vi "Dashboard Main.vi"() -> ()   [LabVIEW 2018]
uses:
  <vilib>/Rock Robotics/Network Tables/NT Read Numeric Array.vi
panel:
  out "Camera Perf":string
  in  "Camera Settings":T1={"Frame Rate"=30, "Compression"=30, "Size"=1, "DB Camera Config"=FALSE} {"Frame Rate" scale=1.0..30.0; "Compression" scale=100.0..-1.0; "Size" items=["640x480", "320x240", "160x120"]}
  in  "TCP":refnum<k5>
  out "Robot IP":string
  in  "Dashboard Tab":enum32{"Drive", "Basic", "Custom", "Variables"}(tab)
  in  "Select Auto":string(combo)="Select Autonomous ..."
  out "NT Connection":bool
  out "MotorChart R":cluster{"Numeric":dbl, "Numeric":dbl}(graph)
  out "MotorChart L":cluster{"Numeric":dbl, "Numeric":dbl}(graph)
  out "MotorSliders R":cluster{"MotorSlide1":dbl, "MotorSlide2":dbl} {"MotorSlide2" scale=-1.0..1.0 scale format="%#_2e"; "MotorSlide1" scale=-1.0..1.0 scale format="%#_2e"}
  out "MotorSliders L":cluster{"MotorSlide1":dbl, "MotorSlide2":dbl} {"MotorSlide2" scale=-1.0..1.0 scale format="%#_2e"; "MotorSlide1" scale=-1.0..1.0 scale format="%#_2e"}
  out "JS1 Z":dbl(slide) scale=-1.0..1.0 scale format="%#_2e"
  out "JS1 Graph":cluster{"X":dbl, "Y":dbl}[](graph)
  out "JS1 Buttons":T2
  out "JS2 Z":dbl(slide) scale=-1.0..1.0 scale format="%#_2e"
  out "JS2 Graph":cluster{"X":dbl, "Y":dbl}[](graph)
  out "JS2 Buttons":T2
  out "Mode":T3(ring)=enum."Auto Disabled"
  in  "DB/String 9":string
  in  "DB/String 8":string
  in  "DB/String 7":string
  in  "DB/String 6":string
  in  "DB/String 5":string
  in  "DB/String 4":string
  in  "DB/String 3":string
  in  "DB/String 2":string
  in  "DB/String 1":string
  in  "DB/String 0":string
  in  "DB/Slider 0":dbl(slide) scale=0.0..5.0
  in  "DB/Slider 1":dbl(slide) scale=0.0..5.0
  in  "DB/Slider 2":dbl(slide) scale=0.0..5.0
  in  "DB/Slider 3":dbl(slide) scale=0.0..5.0
  out "DB/LED 3":bool
  out "DB/LED 2":bool
  out "DB/LED 1":bool
  out "DB/LED 0":bool
  in  "DB/Button 3":bool
  in  "DB/Button 2":bool
  in  "DB/Button 1":bool
  in  "DB/Button 0":bool caption="New Name"
  out "Tree":string(tree)
  out "Camera Image":T4(plugin-control)
  out "Background":bool
  in  "Camera Name":string(combo)="No Camera Selection"
  # "HW"
  # "Joysticks"
  # "Drive Motors"
  # "Front"
  # "Right"
  # "Left"
  # "Back"
  # "This tab is a great place for autonomous settings and robot-specific values.\nPlace controls and indicators inside this tab and match name to\nDashboard Variables on robot. You can also delete this comment."
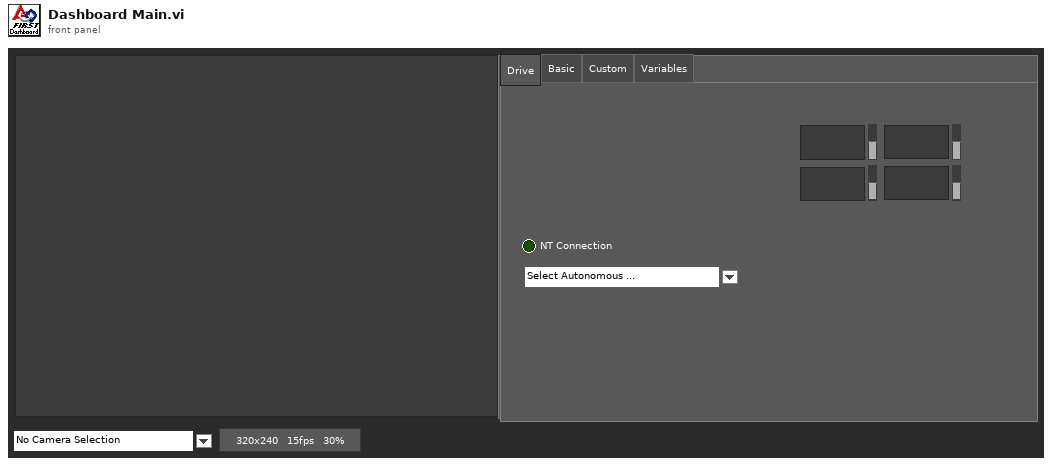
[diagram p1: front panel]
types:
  T1 = cluster{"Frame Rate":i32, "Compression":i32, "Size":u16, "DB Camera Config":bool}
  T2 = cluster{bool, bool, bool, bool, bool, bool, bool, bool, bool, bool, bool, bool}
  T3 = enum8{"Tele-Op Disabled", "Tele-Op Enabled", "Auto Disabled", "Auto Enabled", "Test Disabled", "Test Enabled", "Disconnected", "No Code", "E-Stop"}
  T4 = typedef "IMAQ Image.ctl" = refnum<image>
  T5 = cluster{"Save Path":path, "Interval (s)":dbl, "Keep":i32}
  T6 = typedef "Image Type" = u32
  T7 = cluster{"Camera Image":refnum<vi>, "Dashboard Tab":refnum<vi>, "Background":refnum<vi>, "Tree":refnum<vi>, "Camera Settings":refnum<vi>, "Camera Name":refnum<vi>, "Camera Perf":refnum<vi>}
  T8 = cluster{"Shift":bool, "Ctrl":bool, "Alt":bool, "Cmd":bool, "Opt":bool}
  T9 = cluster{"Error Strings":string, "Disable Counts":cluster{u16, u16}, "Rail Faults":cluster{u16, u16, u16}, "Robot IP":string, "DB Mode":u8, "Event Info":cluster{"Name":string, "Type":u8, "Number":u16, "Replay":u8}}
  T10 = cluster{"Storage":cluster{"Disk Free":u64, "RAM Block":u32, "RAM free":u32}, "CPU Utilization":cluster{"CPU % ISR":sgl, "CPU % Time Crit":sgl, "CPU % Timed Str":sgl, "CPU % High":sgl, "CPU % Above":sgl, "CPU % Normal":sgl, "CPU % Low":sgl}, "CAN":cluster{"% Bus Utilization":sgl, "Bus Off Cnt":u32, "TX_FIFO Full Cnt":u32, "Receive Error Cnt":u8, "Transmit Error Cnt":u8}, "HID":cluster{"HID Outputs":u32, "Rumble Low":u16, "Rumble High":u16}[]}
  T11 = cluster{"Status bits":cluster{"Test Mode":bool, "Autonomous":bool, "Enabled":bool, "Code Start":bool, "Brownout":bool, "Reserved 2":bool, "Reserved 3":bool, "E-Stop":bool}, "Code Trace":cluster{"Disabled":bool, "TeleOp":bool, "Auto":bool, "Test":bool}, "Controller Type":enum16{"unknown", "cRIO", "roboRio"}, "Code?":enum16{"unknown", "noCode", "code"}, "Battery V":dbl}
  T12 = cluster{"Control Bits":cluster{"TestMode":bool, "Autonomous":bool, "Enabled":bool, "FMS Present":bool, bool, bool, bool, "E-Stop":bool}, "Team Station ":u8, "Countdown":sgl, "Joystick Values":cluster{"Axes":dbl[], "Buttons":bool[], "POVs":i16[]}[]}
  T13 = cluster{"Axes":dbl[], "Buttons":bool[], "POVs":i16[]}[]
  T14 = cluster{"Axes":dbl[], "Buttons":bool[], "POVs":i16[]}
  T15 = cluster{"Buttons[0]":bool, "Buttons[1]":bool, "Buttons[2]":bool, "Buttons[3]":bool, "Buttons[4]":bool, "Buttons[5]":bool, "Buttons[6]":bool, "Buttons[7]":bool, "Buttons[8]":bool, "Buttons[9]":bool, "Buttons[10]":bool, "Buttons[11]":bool}
  T16 = cluster{"Camera Name":string, "Camera File Name":string, "Saved DB Images Info":cluster{"Save Path":path, "Interval (s)":dbl, "Keep":i32}}
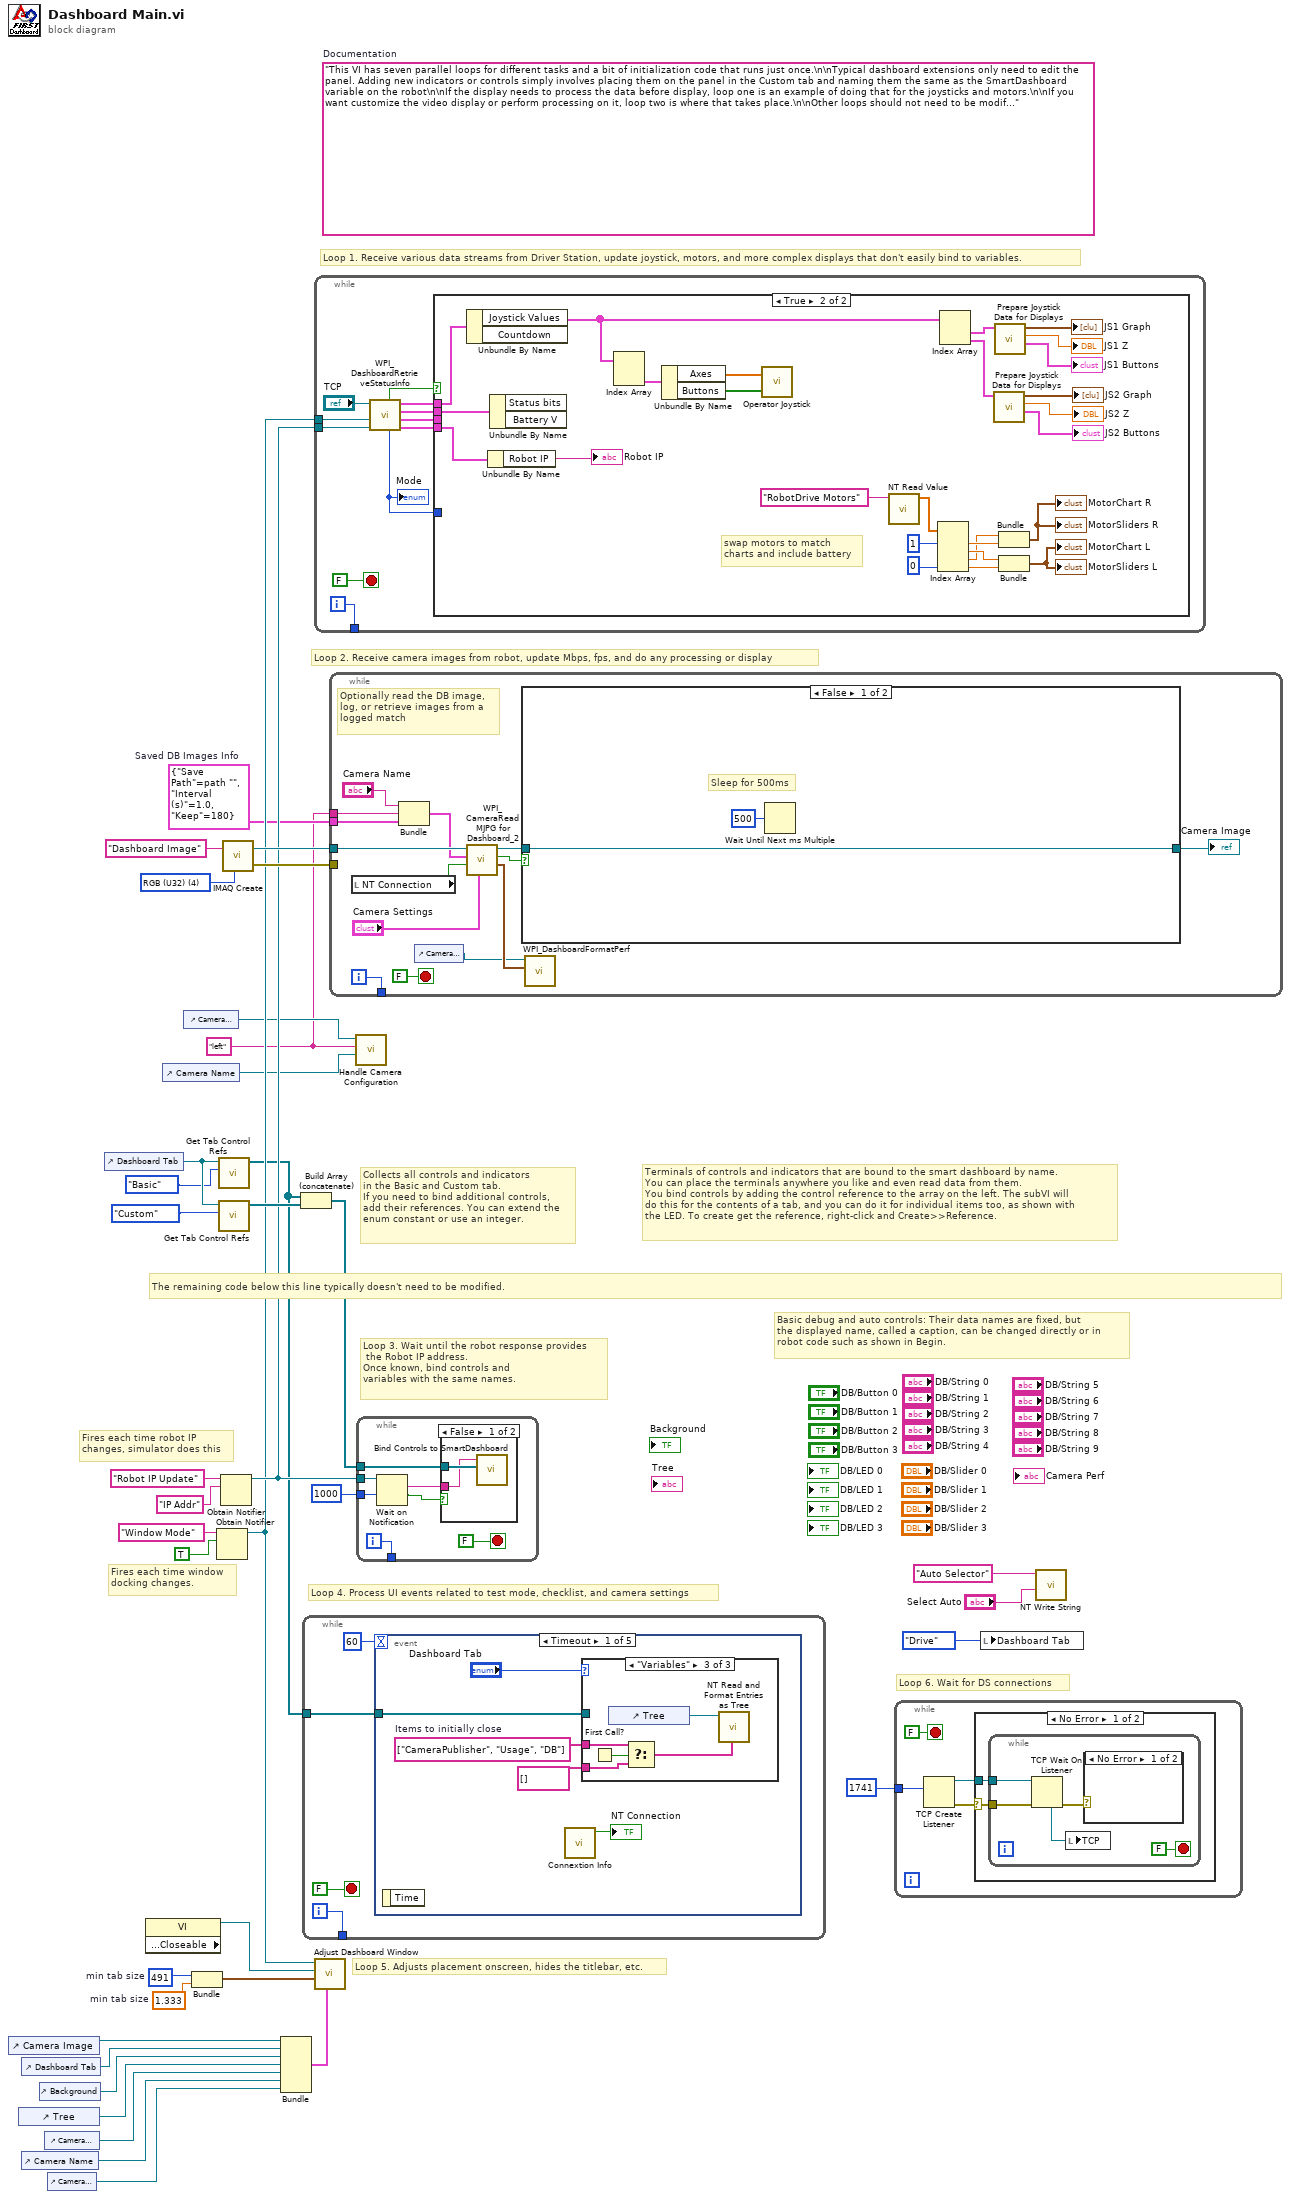
[diagram p0: block diagram]
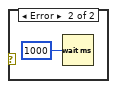
[diagram p2: hidden frame]
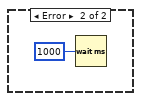
[diagram p3: hidden frame]
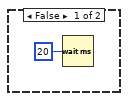
[diagram p4: hidden frame]
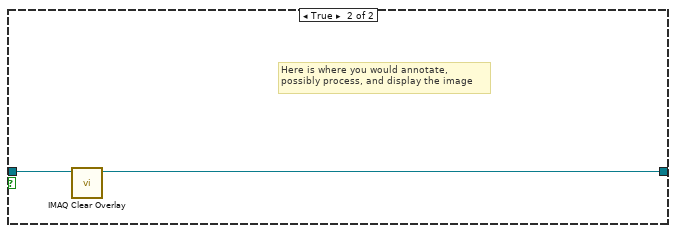
[diagram p6: hidden frame]
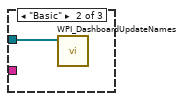
[diagram p8: hidden frame]
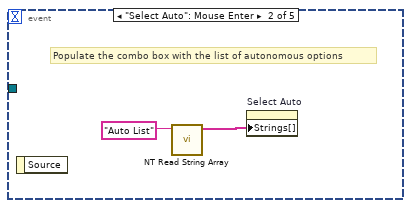
[diagram p9: hidden frame]
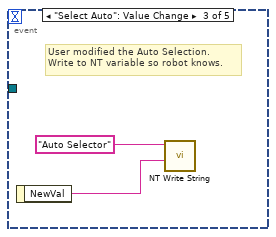
[diagram p10: hidden frame]
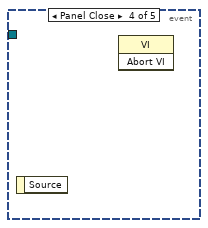
[diagram p11: hidden frame]
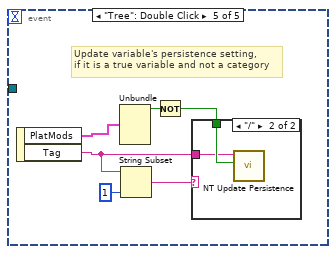
[diagram p12: hidden frame]
diagram:
  w1 = "left" ("Camera File Name")
  w2 = T5 {"Save Path"=path "", "Interval (s)"=1.0, "Keep"=180}  # Saved DB Images Info
  w22 = 491  # min tab size
  w21 = 1.333  # min tab size
  (unwired) "This VI has seven parallel loops for different tasks and a bit of initialization code that runs just once.\n\nTypical dashboard extensions only need to edit the panel. Adding new indicators or controls simply involves placing them on the panel in the Custom tab and naming them the same as the SmartDashboard variable on the robot\n\nIf the display needs to process the data before display, loop one is an example of doing that for the joysticks and motors.\n\nIf you want customize the video display or perform processing on it, loop two is where that takes place.\n\nOther loops should not need to be modified. They are pretty standard, and document the task they perform."  # Documentation
  w37 = T6 4 items=["Grayscale (U8)", "Grayscale (I16)", "Grayscale (SGL)", "Complex (CSG)", "RGB (U32)", "HSL (U32)", "RGB (U64)"] ("Image Type")
  # "Loop 6. Wait for DS connections"
  # "Basic debug and auto controls: Their data names are fixed, but\nthe displayed name, called a caption, can be changed directly or in\nrobot code such as shown in Begin."
  # "Fires each time robot IP\nchanges, simulator does this"
  # "Fires each time window\ndocking changes."
  # "Collects all controls and indicators\nin the Basic and Custom tab.\nIf you need to bind additional controls,\nadd their references. You can extend the\nenum constant or use an integer."
  # "The remaining code below this line typically doesn't need to be modified."
  # "Loop 4. Process UI events related to test mode, checklist, and camera settings"
  # "Terminals of controls and indicators that are bound to the smart dashboard by name.\nYou can place the terminals anywhere you like and even read data from them.\nYou bind controls by adding the control reference to the array on the left. The subVI will\ndo this for the contents of a tab, and you can do it for individual items too, as shown with\nthe LED. To create get the reference, right-click and Create>>Reference."
  # "Loop 3. Wait until the robot response provides\n the Robot IP address.\nOnce known, bind controls and\nvariables with the same names."
  # "Loop 5. Adjusts placement onscreen, hides the titlebar, etc."
  # "Loop 1. Receive various data streams from Driver Station, update joystick, motors, and more complex displays that don't easily bind to variables."
  # "Loop 2. Receive camera images from robot, update Mbps, fps, and do any processing or display"
  n1 = control-ref of="Camera Image"() -> (w24:refnum<vi>)
  n2 = control-ref of="Tree"() -> (w8:refnum<vi>)
  n3 = control-ref of="Dashboard Tab"() -> (w23:refnum<vi>)
  n4 = control-ref of="Camera Name"() -> (w6:refnum<vi>)
  n5 = control-ref of="Background"() -> (w19:refnum<vi>)
  n6 = control-ref of="Camera Settings"() -> (w7:refnum<vi>)
  n7 = control-ref of="Camera Perf"() -> (w5:refnum<vi>)
  n8 = control-ref of="Dashboard Tab"() -> (w27:refnum<vi>)
  n9 = property class="VI" props=["Front Panel.Closeable"]() -> (reference out=w28:refnum<vi>)  [unwired: 2 in, 2 out]
  n10 = control-ref of="Camera Name"() -> (w12:refnum<vi>)
  n11 = control-ref of="Camera Settings"() -> (w13:refnum<vi>)
  n12 = Bundle("min tab size"=w22, "min tab size"=w21) -> (w20:cluster{"min tab size":i32, "min tab size":dbl})  [unwired: 1 in]
  n13 = Obtain Notifier(name (unnamed)="Window Mode", notification data type=TRUE) -> (notifier out=w16:refnum<notifier>)  [unwired: 2 in, 2 out]
  n14 = call <vilib>:"Get Tab Control Refs.vi"("Page Index"=enum32{"Drive", "Basic", "Custom", "Variables"}."Basic" ("Dashboard Tab"), "TabControl in"=w27) -> ("ControlsOnPage"=w11:refnum<vi>[])  [unwired: 9 in]
  n15 = call <vilib>:"Get Tab Control Refs.vi"("Page Index"=enum32{"Drive", "Basic", "Custom", "Variables"}."Custom" ("Dashboard Tab"), "TabControl in"=w27) -> ("ControlsOnPage"=w26:refnum<vi>[])  [unwired: 9 in]
  n16 = Obtain Notifier(name (unnamed)="Robot IP Update", notification data type="IP Addr" ("name (unnamed)")) -> (notifier out=w17:refnum<notifier>)  [unwired: 2 in, 2 out]
  n17 = call "IMAQ Create"("Image Name"="Dashboard Image", "Image Type"=w37) -> ("New Image"=w35:T4, "error out"=w34:errorcluster)  [unwired: 2 in, 1 out]
  n18 = Bundle("Camera Image"=w24, "Dashboard Tab"=w23, "Background"=w19, "Tree"=w8, "Camera Settings"=w7, "Camera Name"=w6, "Camera Perf"=w5) -> (w18:T7)  [unwired: 1 in]
  n19 = Build Array (concatenate)(w11, w26) -> (w25:refnum<vi>[])
  n20 = while {
    tunnel: [w39] -> _
    tunnel: w11 -> [w38]
    i -> [w39]
    stop <- FALSE stop-if-true
    n21 = event shown="[0] Timeout" {
      selector: _ -> [_ _ _ _ _]
      dyn-events: _ -> [_ _ _ _ _]
      timeout: u32 60 ("milliseconds to wait") -> [_ _ _ _ _]
      tunnel: w38 -> [w44 _ _ _ _]
      event Timeout {
        w43 = string[] ["CameraPublisher", "Usage", "DB"]  # Items to initially close
        n22 = event-data() -> ()  [unwired: 1 in, 1 out]
        n23 = call <vilib>:"Connextion Info.vi"() -> ("Connected"=→"NT Connection":bool)  [unwired: 10 in, 1 out]
        n24 = case shown="\"Variables\"" "Dashboard Tab" {
          tunnel: w44 -> [_ w47 _]
          tunnel: w43 -> [_ _ w50]
          tunnel: string[] [] -> [_ _ w49]
          frame "Custom", Default {
          }
          frame "Basic" {
            n25 = call <vilib>:"WPI_DashboardUpdateNames.vi"("Controls on Tab"=w47) -> ()  [unwired: 11 in]
          }
          frame "Variables" {
            n26 = First Call?() -> (First Call?: T/F=w51:bool)
            n27 = control-ref of="Tree"() -> (w52:refnum<vi>)
            n28 = Select(t=w50, s=w51, f=w49) -> (s? t:f=w48:string[])
            n29 = call <vilib>:"NT Read and Format Entries as Tree.vi"("Tags to  Close"=w48, "Tree Refnum"=w52) -> ()  [unwired: 8 in, 2 out]
          }
        }
      }
      event "Select Auto": Mouse Enter {
        # "Populate the combo box with the list of autonomous options"
        n30 = event-data() -> ()  [unwired: 1 in, 1 out]
        n31 = call <vilib>:"NT Read String Array.vi"("Name"="Auto List") -> ("String Array"=w53:string[])  [unwired: 9 in, 1 out]
        n32 = property on="Select Auto" class="CmbBox"("Strings[]"=w53) -> ()  [unwired: 2 in, 2 out]
      }
      event "Select Auto": Value Change {
        # "User modified the Auto Selection.\nWrite to NT variable so robot knows."
        n33 = event-data() -> ("NewVal"=w55:string)  [unwired: 1 in]
        n34 = call <vilib>:"NT Write String.vi"("String"=w55, "Name"="Auto Selector") -> ()  [unwired: 9 in, 1 out]
      }
      event Panel Close {
        n35 = event-data() -> ()  [unwired: 1 in, 1 out]
        n36 = invoke class="VI" method="Abort VI"() -> ()  [unwired: 3 in, 3 out]
      }
      event "Tree": Double Click {
        # "Update variable's persistence setting,\nif it is a true variable and not a category"
        n37 = event-data() -> ("PlatMods"=w58:T8, "Tag"=w57:string)  [unwired: 1 in]
        n38 = Unbundle(w58) -> ("Shift"=w62:bool)  [unwired: 4 out]
        n39 = String Subset(string=w57, length (rest)=1 ("length (rest)")) -> (substring=w59:string)  [unwired: 1 in]
        n40 = Not(x=w62) -> (.not. x?=w61:bool)
        n41 = case shown="\"/\"" w59 {
          tunnel: w61 -> [_ w64]
          tunnel: w57 -> [_ w63]
          frame Default {
          }
          frame "/" {
            n42 = call <vilib>:"NT Update Persistence.vi"("Persistence"=w64, "Name"=w63) -> ()  [unwired: 9 in, 1 out]
          }
        }
      }
    }
  }
  n43 = while {
    tunnel: [w74] -> _
    tunnel: w17 -> [w68]
    tunnel: w16 -> [w65]
    i -> [w74]
    stop <- FALSE stop-if-true
    n44 = call <vilib>:"WPI_DashboardRetrieveStatusInfo.vi"("Binding Refnum"=w68, "Window Mode Notifier"=w65, "TCP Cnx"="TCP") -> ("Power and Errors"=w69:T9, "Robot Metrics"=w72:T10, "Status Info"=w73:T11, "Control Info"=w70:T12, "Robot Mode"=w67:T3, "Process?"=w71:bool)  [unwired: 3 in]
    "Mode" <- w67
    n45 = case shown="True" w71 {
      tunnel: w73 -> [_ w102]
      tunnel: w72 -> [_ _]
      tunnel: w70 -> [_ w101]
      tunnel: w69 -> [_ w100]
      tunnel: w67 -> [_ _]
      frame False {
        n46 = Wait (ms)(milliseconds to wait=u32 20) -> ()  [unwired: 1 out]
      }
      frame True {
        # "swap motors to match\ncharts and include battery"
        n47 = Unbundle By Name(w101) -> ("Joystick Values"=w80:T13)  [unwired: 1 out]
        n48 = Unbundle By Name(w100) -> ("Robot IP"=→"Robot IP":string)
        n49 = Unbundle By Name(w102) -> ()  [unwired: 2 out]
        n50 = Index Array(array=w80) -> (element #2=w79:T14)  [unwired: 2 in, 1 out]
        n51 = Unbundle By Name(w79) -> ("Axes"=w78:dbl[], "Buttons"=w77:bool[])
        n52 = call "Operator Joystick.vi"("Buttons"=w77, "Axes"=w78) -> ()  [unwired: 10 in]
        n53 = call-poly <vilib>:"NT Read Value.vi"("Name"="RobotDrive Motors") -> ("Numeric Array"=w82:dbl[])  [unwired: 9 in, 1 out]
        n54 = Index Array(array=w82, index #1=1, index #4=0) -> (element #1=w95:dbl, element #2=w96:dbl, element #3=w94:dbl, element #4=w99:dbl)  [unwired: 2 in]
        n55 = Index Array(array=w80) -> (element #1=w91:T14, element #2=w87:T14)  [unwired: 2 in]
        n56 = call "Prepare Joystick Data for Displays.vi"("Joystick Values"=w87) -> ("Buttons"=→"JS2 Buttons":T15, "Z Axis"=→"JS2 Z":dbl, "Cartesian Data"=→"JS2 Graph":cluster{"X axis":dbl, "X axis":dbl}[])  [unwired: 8 in]
        n57 = call "Prepare Joystick Data for Displays.vi"("Joystick Values"=w91) -> ("Buttons"=→"JS1 Buttons":T15, "Z Axis"=→"JS1 Z":dbl, "Cartesian Data"=→"JS1 Graph":cluster{"X axis":dbl, "X axis":dbl}[])  [unwired: 8 in]
        n58 = Bundle("Numeric"=w94, "Numeric"=w95) -> (→"MotorChart R" →"MotorSliders R":cluster{"Numeric":dbl, "Numeric":dbl})  [unwired: 1 in]
        n59 = Bundle("Numeric"=w96, "Numeric"=w99) -> (→"MotorChart L" →"MotorSliders L":cluster{"Numeric":dbl, "Numeric":dbl})  [unwired: 1 in]
      }
    }
  }
  n60 = call "Adjust Dashboard Window.vi"("Sizing Refnums"=w18, "Size Constraints"=w20, "VI"=w28, "WIn Mode"=w16) -> ()  [unwired: 8 in]
  n61 = while {
    tunnel: w35 -> [w114]
    tunnel: w34 -> [_]
    tunnel: [w115] -> _
    tunnel: w2 -> [w108]
    tunnel: w1 -> [w105]
    i -> [w115]
    stop <- FALSE stop-if-true
    # "Optionally read the DB image,\nlog, or retrieve images from a\nlogged match"
    n62 = local read "NT Connection"() -> (w109:bool)
    n63 = Bundle("Camera Name"="Camera Name", "Camera File Name"=w105, "Saved DB Images Info"=w108) -> (w107:T16)  [unwired: 1 in]
    n64 = control-ref of="Camera Perf"() -> (w103:refnum<vi>)
    n65 = call <vilib>:"WPI_CameraRead MJPG for Dashboard_2.vi"("Camera Settings"="Camera Settings", "NT Connection"=w109, "Capture Info"=w107, "Image in"=w114) -> ("perf info"=w104:cluster{"Bandwidth (Mbps)":dbl, "fps":dbl}, "Active"=w112:bool, "Image\\ out"=w113:T4)  [unwired: 5 in]
    n66 = case shown="False" w112 {
      tunnel: w113 -> [w117 w120]
      tunnel: [w117 w119] -> w110
      frame False {
        # "Sleep for 500ms"
        n67 = Wait Until Next ms Multiple(millisecond multiple=u32 500) -> ()  [unwired: 1 out]
      }
      frame True {
        # "Here is where you would annotate,\npossibly process, and display the image"
        n68 = call "IMAQ Clear Overlay"("Image"=w120) -> ("Image Out"=w119:T4)  [unwired: 2 in, 8 out]
      }
    }
    "Camera Image" <- w110
    n69 = call <vilib>:"WPI_DashboardFormatPerf.vi"("Performance"=w104, "String in"=w103) -> ()  [unwired: 10 in]
  }
  n70 = call "Handle Camera Configuration.vi"("CameraNameRef"=w12, "Display Name"=w1, "ClusterRef"=w13) -> ()  [unwired: 9 in]
  n71 = while {
    tunnel: w25 -> [w127]
    tunnel: w17 -> [w125]
    tunnel: [w123] -> _
    tunnel: u32 1000 ("milliseconds to wait") -> [w122]
    i -> [w123]
    stop <- FALSE stop-if-true
    n72 = Wait on Notification(notifier=w125, timeout in ms (-1)=w122) -> (notification=w124:string, timed out?=w121:bool)  [unwired: 2 in, 2 out]
    n73 = case shown="False" w121 {
      tunnel: w127 -> [w129 _]
      tunnel: w124 -> [w128 _]
      frame False {
        n74 = call <vilib>:"Bind Controls to SmartDashboard.vi"("Bound Control Refs"=w129, "Server IP Address"=w128) -> ()  [unwired: 10 in]
      }
      frame True {
      }
    }
  }
  n75 = while {
    tunnel: u16 1741 ("timeout ms (25000)") -> [w131]
    stop <- FALSE stop-if-true
    n76 = TCP Create Listener(10:w131) -> (0:w130:errorcluster, 3:w132:refnum<k5>)  [unwired: 4 in, 1 out]
    n77 = case shown="No Error" w130 {
      selector: w130 -> [w134 _]
      tunnel: w132 -> [w135 _]
      frame No Error {
        n78 = while {
          tunnel: w135 -> [w138]
          tunnel: w134 -> [w137]
          stop <- FALSE stop-if-true
          n79 = TCP Wait On Listener(8:w137, 11:w138) -> (0:w139:errorcluster, 4:w140:refnum<k5>)  [unwired: 2 in, 3 out]
          n80 = local write "TCP"(w140) -> ()
          n81 = case shown="No Error" w139 {
            frame No Error {
            }
            frame Error {
              n82 = Wait (ms)(milliseconds to wait=u32 1000) -> ()  [unwired: 1 out]
            }
          }
        }
      }
      frame Error {
        n83 = Wait (ms)(milliseconds to wait=u32 1000) -> ()  [unwired: 1 out]
      }
    }
  }
  n84 = local write "Dashboard Tab"(enum32{"Drive", "Basic", "Custom", "Variables"}."Drive" ("Dashboard Tab")) -> ()
  n85 = call <vilib>:"NT Write String.vi"("String"="Select Auto", "Name"="Auto Selector") -> ()  [unwired: 9 in, 1 out]
